vi "Process.vi"(8 "error in (no error)":errorcluster, 11 "SMO.UI":refnum<class "SMO.UI.lvclass">) -> (0 "error out":errorcluster, 3 "SMO.UI out":refnum<class "SMO.UI.lvclass">)   [LabVIEW 2021, in "smo.lvlib" / "SMO.UI.lvclass"]
uses:
  SMO.UI.lvclass
  C:/Repositories/SMO/src/SMO/SMO.lvclass
  SMO/Typedefs/Parent Call--Enum.ctl
  SMO/SMO.lvclass
  SMO/SMO.lvclass/SMO.ctl
  SMO.UI.lvclass/SMO.UI.ctl
  Typedefs/SMO.UI State--enum.ctl
  SMO/Private/GetVariant(Attr).vi
  Support/Attribute.Identity/Read UniqueName.vi
  Support/Attribute.Identity/Read Given Name.vi
  Support/Attribute.Identity/Read ProspectiveOwner.vi
  SMO/Private/ReftoDVR--SMO.vi
  SMO.UI.ReftoDVR.vi
  Support/Attribute.Identity/Attribute.Identity.lvclass
panel:
  in  "self terminate":bool
  out "Copyright":string="JKI State Machine Objects™\nhttp://jki.net/state-machine-objects/\nCopyright (C) 2005-2015, JKI <info@jki.net>\nALL RIGHTS RESERVED\n\nFor instructions on how to use the JKI State Machine Objects, examples and video tutorials, visit:\nhttp://jki.net/state-machine-objects/\n"
  # "JKI SMO UI"
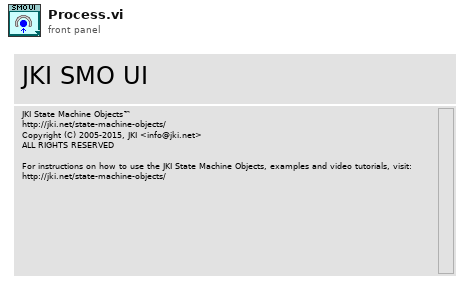
[diagram p1: front panel]
types:
  T1 = typedef "smo.lvlib/SMO.lvclass/Parent Call--Enum.ctl" = enum16{"Allows parent to run", "Does not request parent to run"}
  T2 = enum32{"invalid app kind", "Development System", "Run Time System", "Student Edition", "Embedded LabVIEW", "Evaluation", "Custom"}
  T3 = enum32{"Invalid", "Standard", "Closed", "Hidden", "Minimized", "Maximized"}
  T4 = typedef "smo.lvlib/SMO.UI.lvclass/SMO.UI State--enum.ctl" = enum16{"unknown", "Opened", "Closed"}
  T5 = cluster{"Core":cluster{"Current VI Reference":refnum<vi>, "Close Panel on Exit?":bool, "Last Error":cluster{"error":errorcluster, "previous state":string, "remaining states":string}}, "SMO out":refnum<class "SMO.UI.lvclass">}
  T6 = cluster{"Current VI Reference":refnum<vi>, "Close Panel on Exit?":bool, "Last Error":cluster{"error":errorcluster, "previous state":string, "remaining states":string}}
  T7 = typedef "smo.lvlib/SMO.lvclass/Protected Events.ctl" = cluster{"StopProcesses":refnum<user-event>, "AbortProcesses":refnum<user-event>, "Config Changed":refnum<user-event>, "Dependency":refnum<user-event>}
  T8 = typedef "smo.lvlib/SMO.UI.lvclass/PrivateEvents--Cluster.ctl" = cluster{"Show-Hide UI":refnum<user-event>}
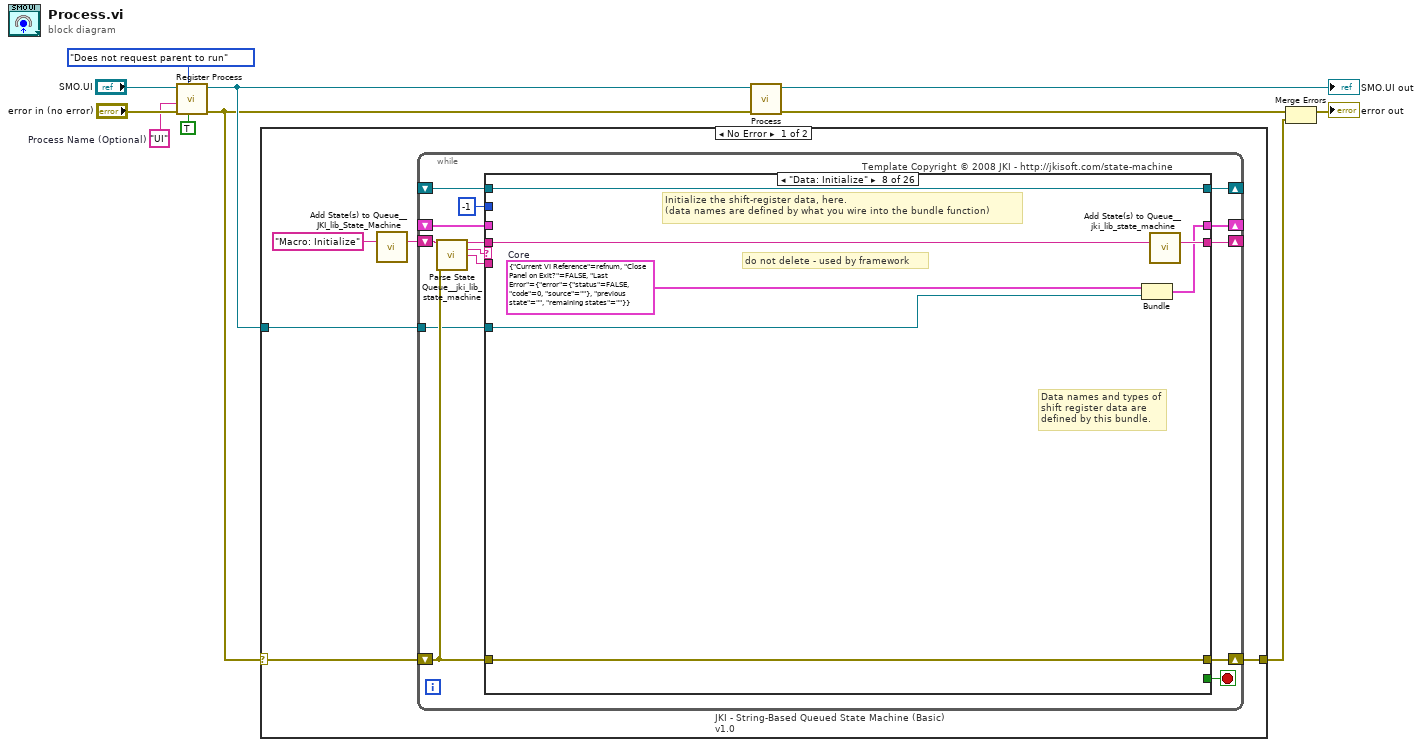
[diagram p0: block diagram]
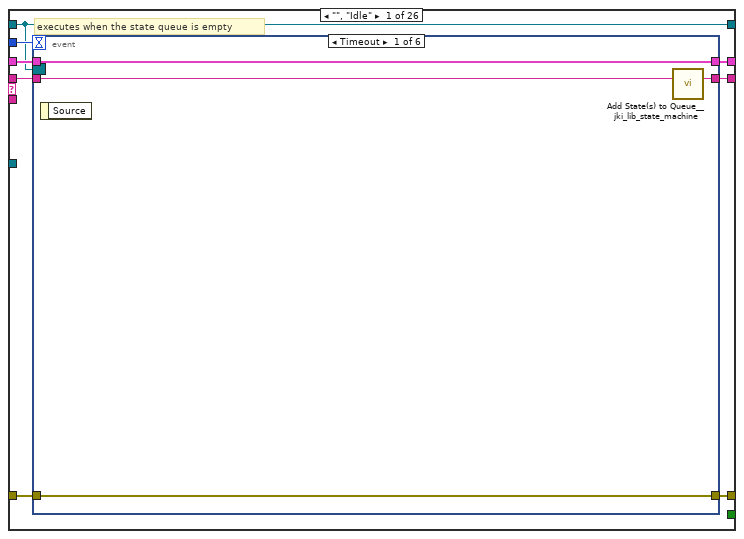
[diagram p2: hidden frame]
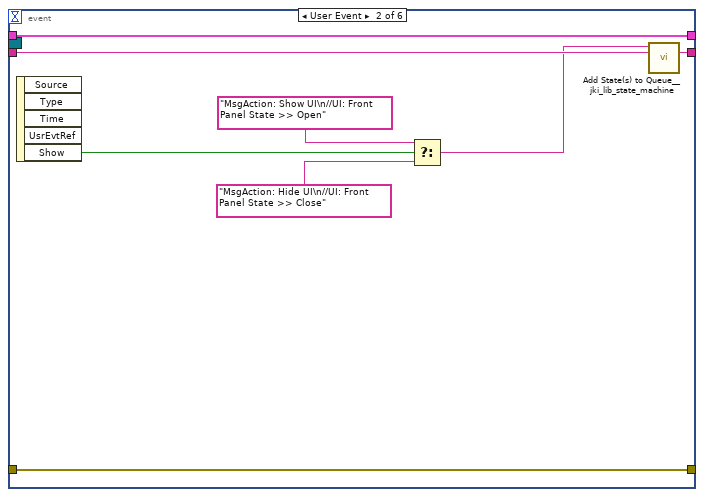
[diagram p3: hidden frame]
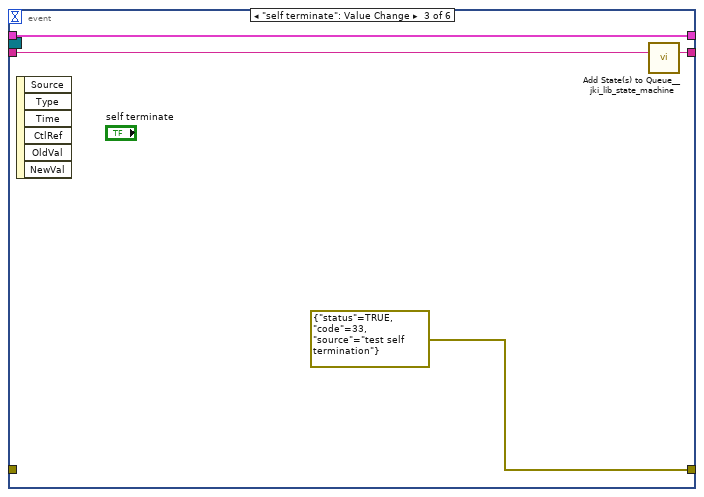
[diagram p4: hidden frame]
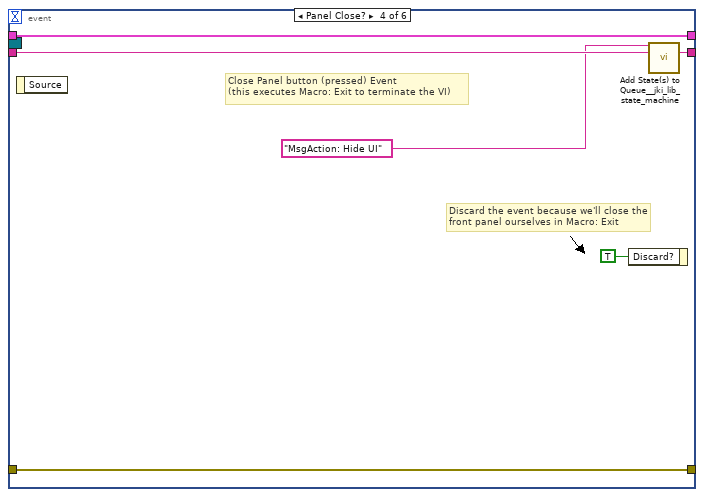
[diagram p5: hidden frame]
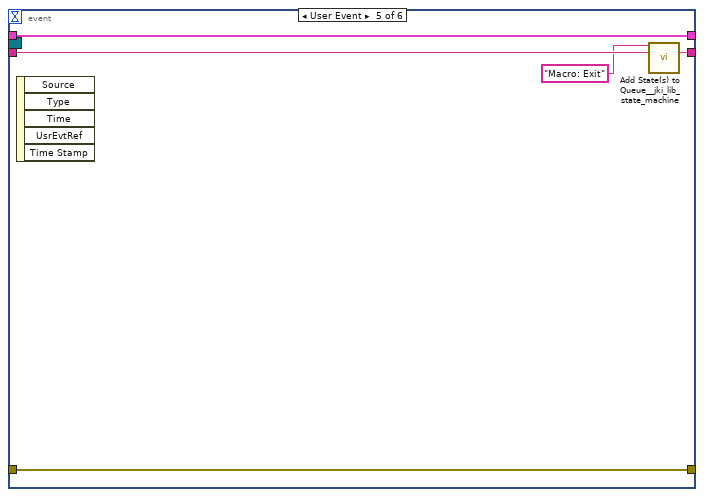
[diagram p6: hidden frame]
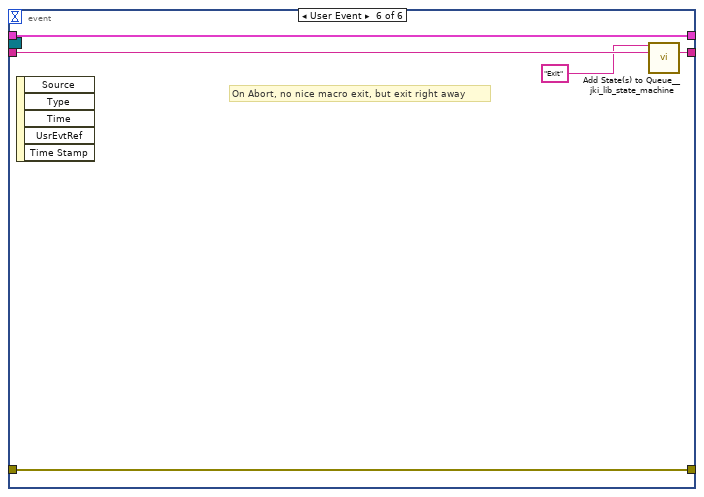
[diagram p7: hidden frame]
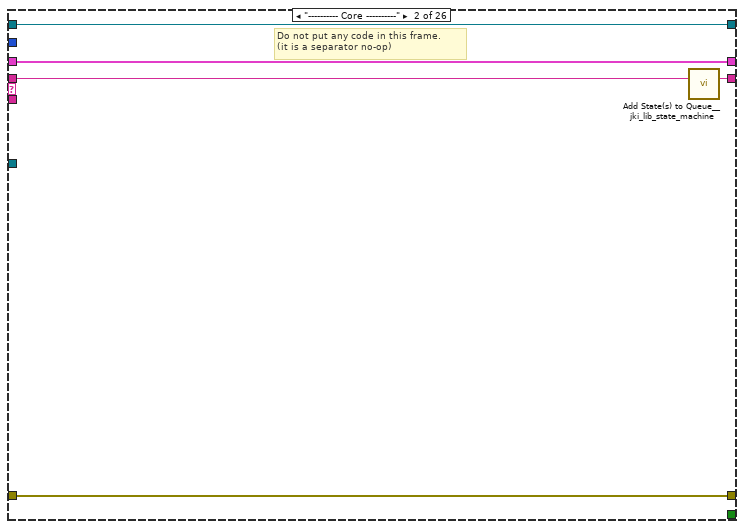
[diagram p8: hidden frame]
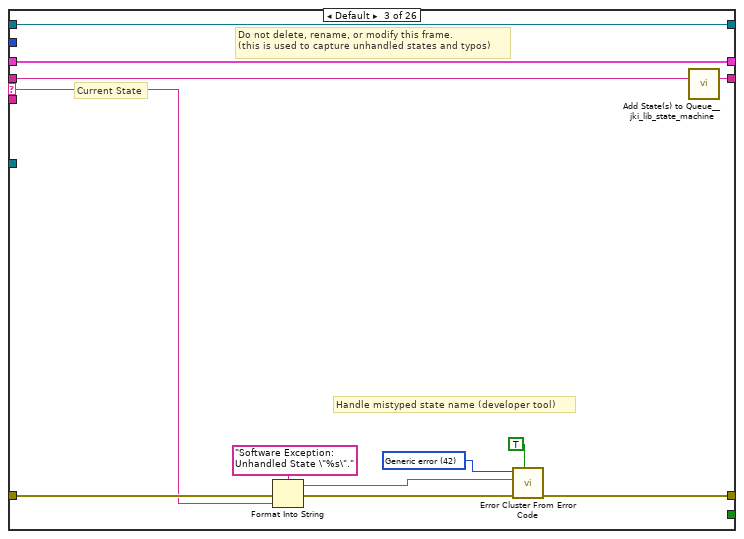
[diagram p9: hidden frame]
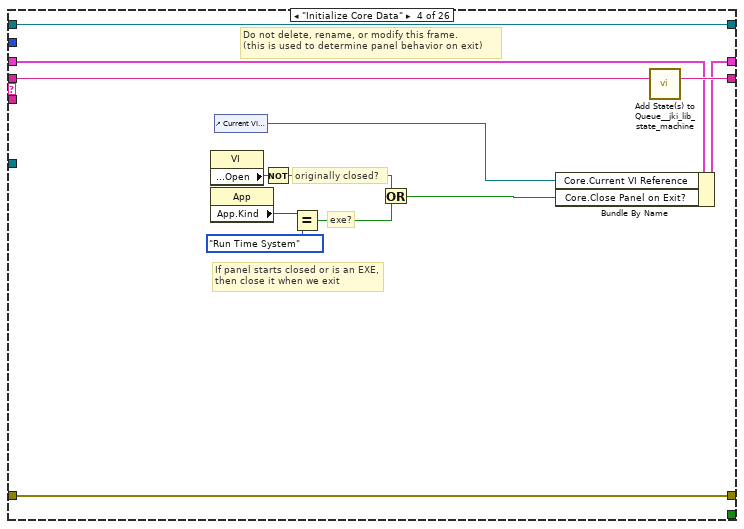
[diagram p10: hidden frame]
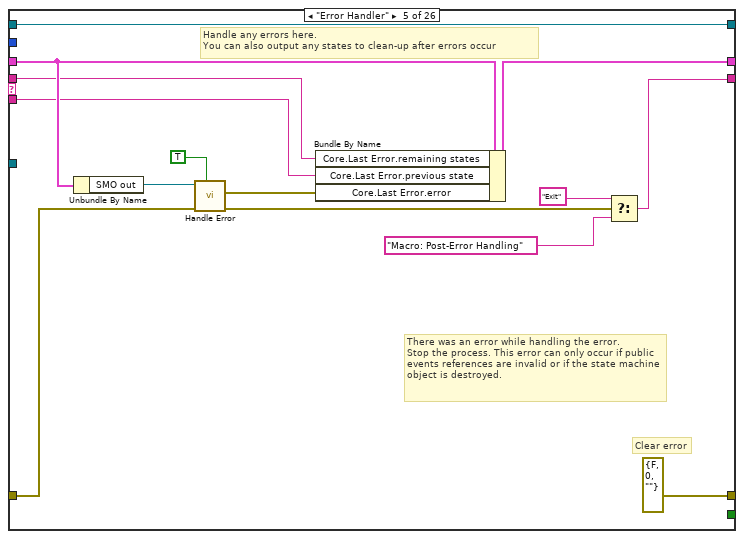
[diagram p11: hidden frame]
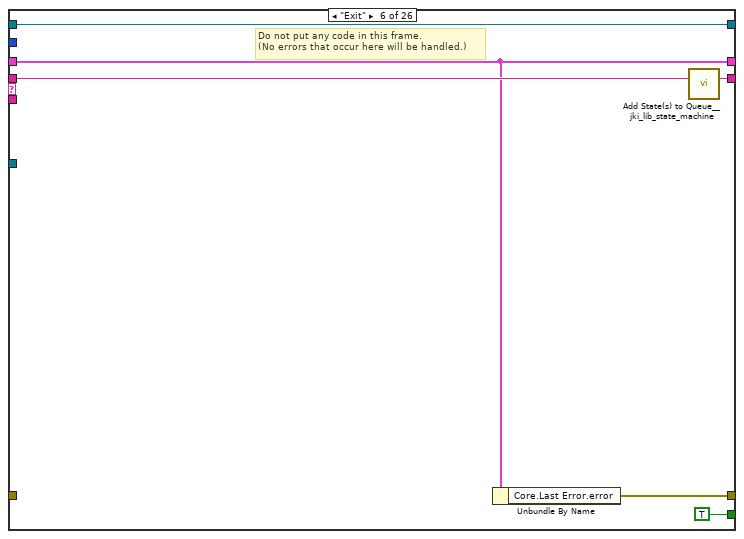
[diagram p12: hidden frame]
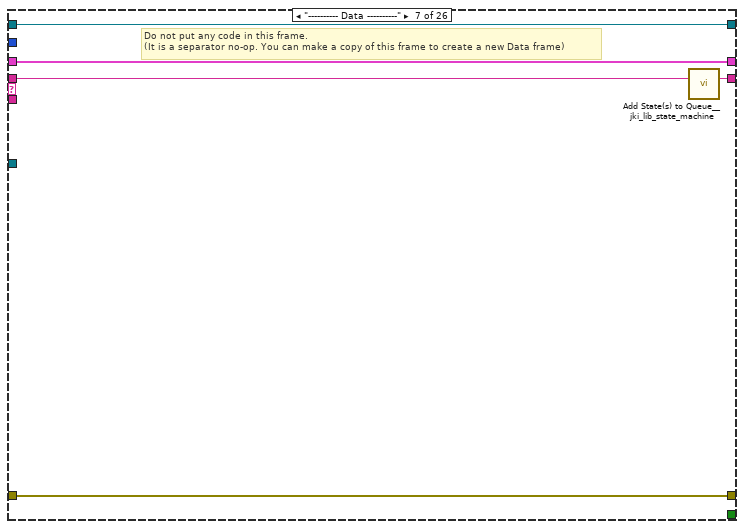
[diagram p13: hidden frame]
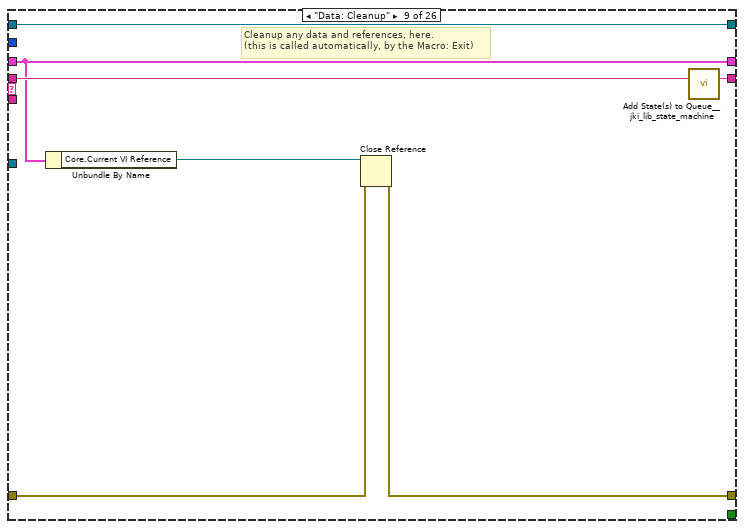
[diagram p14: hidden frame]
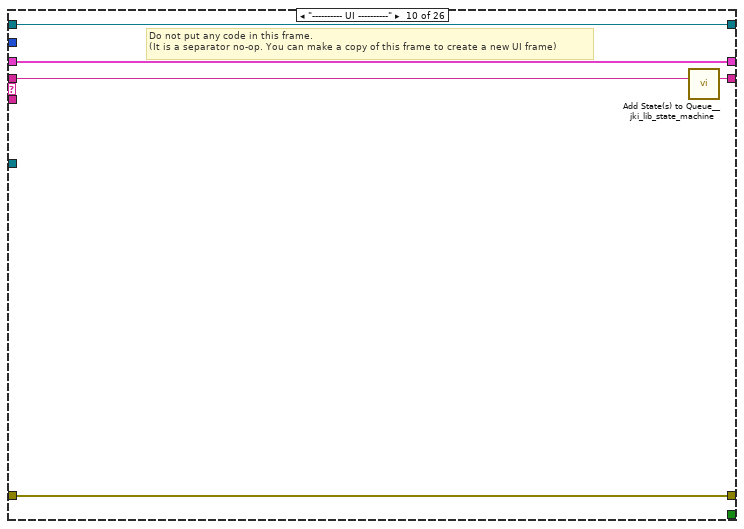
[diagram p15: hidden frame]
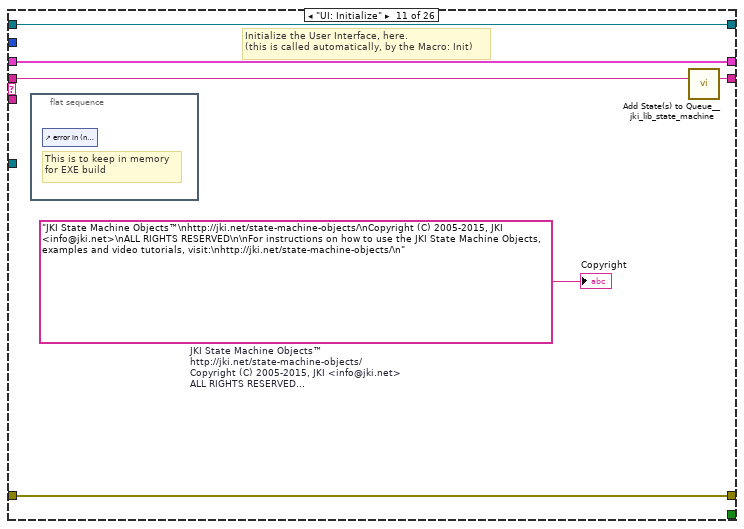
[diagram p16: hidden frame]
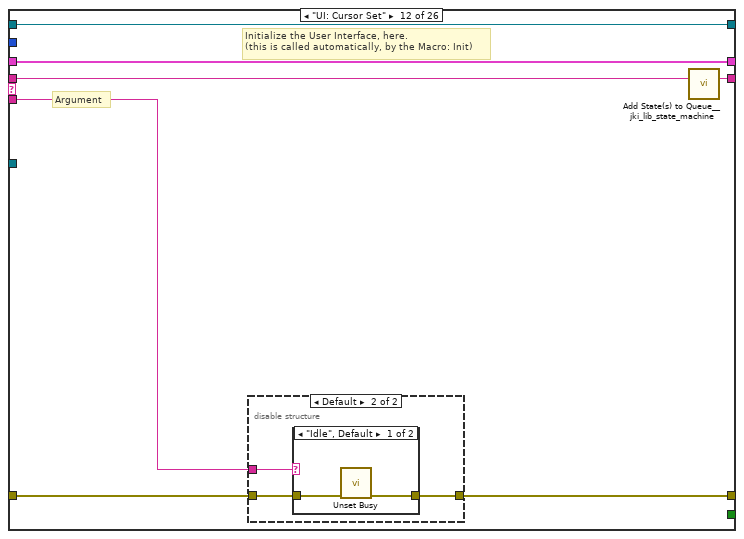
[diagram p17: hidden frame]
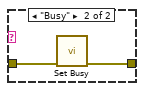
[diagram p19: hidden frame]
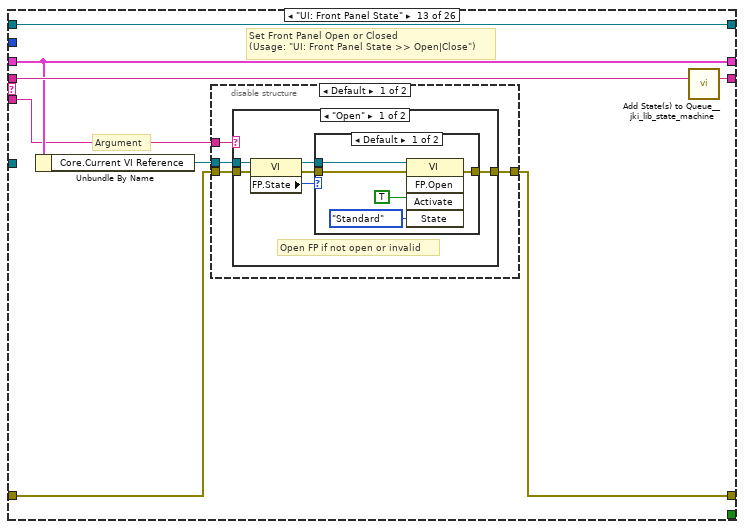
[diagram p20: hidden frame]
diagram:
  w4 = "UI"  # Process Name (Optional)
  n1 = call "Register Process.vi"("Forces Self to Run (F)"=TRUE, "Parent Call"=Parent_Call--Enum."Does not request parent to run", "error in (no error)"="error in (no error)", "Process Name (optional)"=w4, "SMO"="SMO.UI") -> ("error out"=w10:errorcluster, "SMO out"=w11:refnum<class "SMO.UI.lvclass">)  [unwired: 5 in]
  n2 = case shown="No Error" w10 {
    selector: w10 -> [w15 w324]
    tunnel: w11 -> [w16 _]
    tunnel: [w14 w324] -> w8
    frame No Error {
      n3 = call <vilib>:"Add State(s) to Queue__JKI_lib_State_Machine.vi"("State(s) in (\"\")"="Macro: Initialize") -> ("States Out"=w12:string)  [unwired: 14 in]
      n4 = while "JKI - String-Based Queued State Machine (Basic) v1.0" {
        shift-right: [w23] -> _
        shift-left: _ -> [w22]
        shift-right: [w26] -> w14
        shift-left: w15 -> [w20]
        shift-right: [w25] -> _
        shift-left: w12 -> [w27]
        tunnel: w16 -> [w19]
        shift-right: [w18] -> _
        shift-left: _ -> [w17]
        stop <- w24 stop-if-true
        # "Template Copyright © 2008 JKI - http://jkisoft.com/state-machine"
        n5 = call <vilib>:"Parse State Queue__jki_lib_state_machine.vi"("State Queue"=w27, "Error In (no error)"=w20) -> ("Remaining States"=w29:string, "Current State"=w30:string, "Arguments"=w28:string)  [unwired: 11 in]
        n6 = case shown="\"Data: Initialize\"" w30 {
          selector: w30 -> [_ _ w77 _ _ _ _ _ _ _ _ _ _ _ _ _ _ _ _ _ _ _ _ _ _ _]
          tunnel: w29 -> [w38 w75 w81 w100 w102 w120 w125 w132 w139 w144 w150 w157 w173 w205 w214 w223 w235 w240 w251 w263 w268 w280 w286 w291 w301 w316]
          tunnel: w28 -> [_ _ _ _ w103 _ _ _ _ _ _ w151 w169 _ _ _ _ _ _ _ _ _ _ _ _ _]
          tunnel: w22 -> [w36 w72 w79 w91 w112 w116 w122 _ w134 w141 w148 w155 w171 w202 w210 w219 w226 w237 w248 w260 w265 w278 w284 w288 w298 w313]
          tunnel: [w35 w73 w83 w97 errorcluster {"status"=FALSE, "code"=0, "source"=""} ("error out") w115 w123 w126 w135 w142 w147 w152 w166 w203 w212 w221 w233 w238 w242 w258 w266 w276 w282 w289 w292 w307] -> w26
          tunnel: w20 -> [w34 w73 w82 w97 w109 _ w123 w126 w136 w142 w147 w153 w167 w203 w212 w221 w233 w238 w243 w255 w266 w269 w282 w289 w296 w311]
          tunnel: [w37 w74 w80 w99 w101 w119 w124 w131 w138 w143 w149 w156 w172 w204 w213 w222 w234 w239 w250 w262 w267 w279 w285 w290 w300 w315] -> w25
          tunnel: [_ _ _ _ _ TRUE _ _ _ _ _ _ _ _ _ _ _ _ _ _ _ _ _ _ _ _] -> w24
          tunnel: [w33 w72 w79 w98 w111 w116 w122 w130 w134 w141 w148 w155 w171 w202 w210 w218 w226 w237 w248 w260 w265 w278 w284 w288 w298 w313] -> w23
          tunnel: -1 ("Timeout") -> [w32 _ _ _ _ _ _ _ _ _ _ _ _ _ _ _ _ _ _ _ _ _ _ _ _ _]
          tunnel: w19 -> [_ _ _ _ _ _ _ w127 _ _ _ _ _ _ _ _ _ _ _ _ _ _ _ _ _ _]
          tunnel: [w31 w71 w76 w88 w114 w117 w121 w129 w133 w140 w146 w154 w170 w201 w211 w220 w227 w236 w249 w261 w264 w275 w283 w287 w299 w314] -> w18
          tunnel: w17 -> [w31 w71 w76 w88 w114 w117 w121 w129 w133 w140 w146 w154 w170 w201 w211 w220 w227 w236 w249 w261 w264 _ w283 w287 w299 w314]
          frame "", "Idle" {
            # "executes when the state queue is empty"
            n7 = event shown="[0] Timeout" {
              selector: w31 -> [_ _ _ _ _ _]
              dyn-events: _ -> [_ _ _ _ _ _]
              timeout: w32 -> [_ _ _ _ _ _]
              tunnel: w38 -> [w42 w50 w54 w60 w65 w70]
              tunnel: [w41 w49 w53 w59 w64 w69] -> w37
              tunnel: w36 -> [w39 w47 w52 w56 w62 w67]
              tunnel: [w40 w48 errorcluster {"status"=TRUE, "code"=33, "source"="test self termination"} ("error IO") w58 w63 w68] -> w35
              tunnel: w34 -> [w40 w48 _ w58 w63 w68]
              tunnel: [w39 w47 w52 w56 w62 w67] -> w33
              event Timeout {
                n8 = event-data() -> ()  [unwired: 1 in, 1 out]
                n9 = call <vilib>:"Add State(s) to Queue__jki_lib_state_machine.vi"("State(s) in (\"\")"=w42) -> ("States Out"=w41:string)  [unwired: 14 in]
              }
              event User Event {
                n10 = event-data() -> ("Show"=w46:bool)  [unwired: 1 in, 4 out]
                n11 = Select(t="MsgAction: Show UI\n//UI: Front Panel State >> Open" ("State(s) in Front (\"\")"), s=w46, f="MsgAction: Hide UI\n//UI: Front Panel State >> Close" ("State(s) in Front (\"\")")) -> (s? t:f=w43:string)
                n12 = call <vilib>:"Add State(s) to Queue__jki_lib_state_machine.vi"("State(s) in Front (\"\")"=w43, "State(s) in (\"\")"=w50) -> ("States Out"=w49:string)  [unwired: 13 in]
              }
              event "self terminate": Value Change {
                n13 = event-data() -> ()  [unwired: 1 in, 6 out]
                n14 = call <vilib>:"Add State(s) to Queue__jki_lib_state_machine.vi"("State(s) in (\"\")"=w54) -> ("States Out"=w53:string)  [unwired: 14 in]
              }
              event Panel Close? {
                # "Discard the event because we'll close the front panel ourselves in Macro: Exit"
                # "Close Panel button (pressed) Event\n(this executes Macro: Exit to terminate the VI)"
                n15 = event-data() -> ()  [unwired: 1 in, 1 out]
                n16 = event-data("Discard?"=TRUE) -> ()  [unwired: 1 in, 1 out]
                n17 = call <vilib>:"Add State(s) to Queue__jki_lib_state_machine.vi"("State(s) in Front (\"\")"="MsgAction: Hide UI", "State(s) in (\"\")"=w60) -> ("States Out"=w59:string)  [unwired: 13 in]
              }
              event User Event {
                n18 = event-data() -> ()  [unwired: 1 in, 5 out]
                n19 = call <vilib>:"Add State(s) to Queue__jki_lib_state_machine.vi"("State(s) in Front (\"\")"="Macro: Exit", "State(s) in (\"\")"=w65) -> ("States Out"=w64:string)  [unwired: 13 in]
              }
              event User Event {
                # "On Abort, no nice macro exit, but exit right away"
                n20 = event-data() -> ()  [unwired: 1 in, 5 out]
                n21 = call <vilib>:"Add State(s) to Queue__jki_lib_state_machine.vi"("State(s) in Front (\"\")"="Exit", "State(s) in (\"\")"=w70) -> ("States Out"=w69:string)  [unwired: 13 in]
              }
            }
          }
          frame "---------- Core ----------" {
            # "Do not put any code in this frame.\n(it is a separator no-op)"
            n22 = call <vilib>:"Add State(s) to Queue__jki_lib_state_machine.vi"("State(s) in (\"\")"=w75) -> ("States Out"=w74:string)  [unwired: 14 in]
          }
          frame Default {
            w86 = 42 items=["No error", "Argument error", "Memory is full", "Out of zone", "End of file", "File already open", "Generic file I/O error", "File not found", "File permission error", "Disk is full", "Duplicate path", "Too many files open", "System feature not enabled", "Resource file not found", "Cannot add resource", "Resource not found", "Image not found", "Image memory error", "Pen does not exist", "Config type invalid", "Config token not found", "Config parse error", "Config memory error", "Bad external code format", "Bad external code offset", "External code not present", "Null window", "Destroy window error", "Null menu", "Print aborted", "Bad print record", "Print driver error", "Windows error during printing", "Memory error during printing", "Print dialog error", "Generic print error", "Invalid device refnum", "Device not found", "Device parameter error", "Device unit error", "Cannot open device", "Device call aborted", "Generic error", "Cancelled by user", "Object ID too low", "Object ID too high", "Object not in heap", "Unknown heap", "Unknown object (invalid DefProc)", "Unknown object (DefProc not in table)", "Message out of range", "Invalid (null) method", "Unknown message", "Manager call not supported", "Bad address", "Network operation in progress", "Network operation timed out", "Connection is busy", "Network attribute not supported", "Network error", "Address in use", "System out of memory", "Connection aborted", "Connection refused", "Not connected", "Already connected", "Connection closed", "Initialization error (interapplication manager)", "Bad occurrence", "Wait on unbound occurrence handler", "Occurrence queue overflow", "Datalog type conflict", "Unused", "Unrecognized type (interapplication manager)", "Memory corrupt", "Failed to make temporary DLL", "Old CIN version", "Drag socket not found", "Failed to load drop-object", "Failed to register OLE object", "Failed to release OLE object", "Format specifier type mismatch", "Unknown format specifier", "Too few format specifiers", "Too many format specifiers", "Scan failed", "Newer CIN version", "Error converting to variant", "Runtime menu error", "Password tampered", "Variant attribute not found", "Incompatible variant data type", "Event data is not available", "Event Store is not present", "Occurrence is not found", "Event Queue is not created", "Event info is not available", "Refnum passed is NULL", "Error retrieving Class GUID", "Error retrieving CoClass GUID", "Error retrieving TypeLib GUID.", "Bad built application magic bytes.", "Specific driver is different from the specific driver associated with the Logical Name.", "There is no session opened to the class driver.", "Max Error", "MAX - Error with config objects", "MAX - Error loading configuration", "MAX - Group not supported"]
            # "Current State"
            # "Do not delete, rename, or modify this frame.\n(this is used to capture unhandled states and typos)"
            # "Handle mistyped state name (developer tool)"
            n23 = Format Into String(format string="Software Exception: Unhandled State \"%s\"." ("message"), error in=w82, w77) -> (resulting string=w85:string, error out=w84:errorcluster)  [unwired: 1 in]
            n24 = call <vilib>:"Error Cluster From Error Code.vi"("show call chain? (False)"=TRUE, "error in (no error)"=w84, "error message (\"\")"=w85, "error code (0)"=w86) -> ("error out"=w83:errorcluster)  [unwired: 5 in]
            n25 = call <vilib>:"Add State(s) to Queue__jki_lib_state_machine.vi"("State(s) in (\"\")"=w81) -> ("States Out"=w80:string)  [unwired: 14 in]
          }
          frame "Initialize Core Data" {
            # "Do not delete, rename, or modify this frame.\n(this is used to determine panel behavior on exit)"
            # "originally closed?"
            # "exe?"
            # "If panel starts closed or is an EXE, then close it when we exit"
            n26 = property class="VI"() -> ("Front Panel.Open"=w96:bool)  [unwired: 2 in, 2 out]
            n27 = property class="App"() -> ("App.Kind"=w95:T2)  [unwired: 2 in, 2 out]
            n28 = control-ref of="Current VI Reference"() -> (w89:refnum<vi>)
            n29 = Not(x=w96) -> (.not. x?=w93:bool)
            n30 = Equal?(x=w95, y=T2."Run Time System" ("Application:Kind")) -> (x = y?=w92:bool)
            n31 = Or(x=w93, y=w92) -> (x .or. y?=w90:bool)
            n32 = Bundle By Name(cluster=w91, "Core.Current VI Reference"=w89, "Core.Close Panel on Exit?"=w90) -> (w98:T5)
            n33 = call <vilib>:"Add State(s) to Queue__jki_lib_state_machine.vi"("State(s) in (\"\")"=w100) -> ("States Out"=w99:string)  [unwired: 14 in]
          }
          frame "Error Handler" {
            # "There was an error while handling the error.\nStop the process. This error can only occur if public events references are invalid or if the state machine object is destroyed."
            # "Handle any errors here.\nYou can also output any states to clean-up after errors occur"
            # "Clear error"
            n34 = Unbundle By Name(w112) -> ("SMO out"=w113:refnum<class "SMO.UI.lvclass">)
            n35 = call-dynamic "Handle Error.vi"("Stop on Unhandled Error (T)"=TRUE, "error in"=w109, "SMO"=w113) -> ("handling error"=w107:errorcluster, "Unhandled error"=w110:errorcluster)  [unwired: 6 in, 1 out]
            n36 = Bundle By Name(cluster=w112, "Core.Last Error.remaining states"=w102, "Core.Last Error.previous state"=w103, "Core.Last Error.error"=w110) -> (w111:T5)
            n37 = Select(t="Exit", s=w107, f="Macro: Post-Error Handling") -> (s? t:f=w101:string)
          }
          frame "Exit" {
            # "Do not put any code in this frame.\n(No errors that occur here will be handled.)"
            n38 = Unbundle By Name(w116) -> ("Core.Last Error.error"=w115:errorcluster)
            n39 = call <vilib>:"Add State(s) to Queue__jki_lib_state_machine.vi"("State(s) in (\"\")"=w120) -> ("States Out"=w119:string)  [unwired: 14 in]
          }
          frame "---------- Data ----------" {
            # "Do not put any code in this frame.\n(It is a separator no-op. You can make a copy of this frame to create a new Data frame)"
            n40 = call <vilib>:"Add State(s) to Queue__jki_lib_state_machine.vi"("State(s) in (\"\")"=w125) -> ("States Out"=w124:string)  [unwired: 14 in]
          }
          frame "Data: Initialize" {
            w128 = T6 {"Current VI Reference"=refnum, "Close Panel on Exit?"=FALSE, "Last Error"={"error"={"status"=FALSE, "code"=0, "source"=""}, "previous state"="", "remaining states"=""}}  # Core
            # "do not delete - used by framework"
            # "Data names and types of shift register data are defined by this bundle."
            # "Initialize the shift-register data, here.\n(data names are defined by what you wire into the bundle function)"
            n41 = Bundle("Core"=w128, "SMO out"=w127) -> (w130:T5)  [unwired: 1 in]
            n42 = call <vilib>:"Add State(s) to Queue__jki_lib_state_machine.vi"("State(s) in (\"\")"=w132) -> ("States Out"=w131:string)  [unwired: 14 in]
          }
          frame "Data: Cleanup" {
            # "Cleanup any data and references, here.\n(this is called automatically, by the Macro: Exit)"
            n43 = Unbundle By Name(w134) -> ("Core.Current VI Reference"=w137:refnum<vi>)
            n44 = Close Reference(reference=w137, error in (no error)=w136) -> (error out=w135:errorcluster)
            n45 = call <vilib>:"Add State(s) to Queue__jki_lib_state_machine.vi"("State(s) in (\"\")"=w139) -> ("States Out"=w138:string)  [unwired: 14 in]
          }
          frame "---------- UI ----------" {
            # "Do not put any code in this frame.\n(It is a separator no-op. You can make a copy of this frame to create a new UI frame)"
            n46 = call <vilib>:"Add State(s) to Queue__jki_lib_state_machine.vi"("State(s) in (\"\")"=w144) -> ("States Out"=w143:string)  [unwired: 14 in]
          }
          frame "UI: Initialize" {
            w145 = "JKI State Machine Objects™\nhttp://jki.net/state-machine-objects/\nCopyright (C) 2005-2015, JKI <info@jki.net>\nALL RIGHTS RESERVED\n\nFor instructions on how to use the JKI State Machine Objects, examples and video tutorials, visit:\nhttp://jki.net/state-machine-objects/\n"  # JKI State Machine Objects™ http://jki.net/state-machine-objects/ Copyright (C) 2005-2015, JKI <info@jki.net> ALL RIGHTS RESERVED  For instructions on how to use the JKI State Machine Objects, examples and video tutorials, visit: http://jki.net/state-machine-objects/
            # "Initialize the User Interface, here.\n(this is called automatically, by the Macro: Init)"
            n47 = flat-sequence {
              frame #0 {
                # "This is to keep in memory\nfor EXE build"
                n48 = control-ref of="error in (no error)"() -> ()  [unwired: 1 out]
              }
            }
            n49 = call <vilib>:"Add State(s) to Queue__jki_lib_state_machine.vi"("State(s) in (\"\")"=w150) -> ("States Out"=w149:string)  [unwired: 14 in]
            "Copyright" <- w145
          }
          frame "UI: Cursor Set" {
            # "Argument"
            # "Initialize the User Interface, here.\n(this is called automatically, by the Macro: Init)"
            n50 = disable-structure shown="Default" {
              disable-tunnel: w153 -> [w158 w161]
              disable-tunnel: [w158 w160] -> w152
              disable-tunnel: w151 -> [_ w159]
              frame condition #0 {
              }
              frame condition #1 (active) {
                n51 = case shown="\"Idle\", Default" w159 {
                  tunnel: w161 -> [w163 w165]
                  tunnel: [w162 w164] -> w160
                  frame "Idle", Default {
                    n52 = call <vilib>:"Unset Busy.vi"("error in (no error)"=w163) -> ("error out"=w162:errorcluster)  [unwired: 10 in]
                  }
                  frame "Busy" {
                    n53 = call <vilib>:"Set Busy.vi"("error in (no error)"=w165) -> ("error out"=w164:errorcluster)  [unwired: 9 in, 1 out]
                  }
                }
              }
            }
            n54 = call <vilib>:"Add State(s) to Queue__jki_lib_state_machine.vi"("State(s) in (\"\")"=w157) -> ("States Out"=w156:string)  [unwired: 14 in]
          }
          frame "UI: Front Panel State" {
            # "Argument"
            # "Set Front Panel Open or Closed\n(Usage: \"UI: Front Panel State >> Open|Close\")"
            n55 = Unbundle By Name(w171) -> ("Core.Current VI Reference"=w168:refnum<vi>)
            n56 = disable-structure shown="Default" {
              disable-tunnel: w167 -> [w177 w200]
              disable-tunnel: [w176 w200] -> w166
              disable-tunnel: w168 -> [w175 _]
              disable-tunnel: w169 -> [w174 _]
              frame condition #0 (active) {
                n57 = case shown="\"Open\"" w174 {
                  tunnel: w177 -> [w181 w194]
                  tunnel: [w183 w195] -> w176
                  tunnel: w175 -> [w182 w192]
                  frame "Open" {
                    # "Open FP if not open or invalid"
                    n58 = property class="VI"(reference=w182, error in=w181) -> (reference out=w179:refnum<vi>, error out=w180:errorcluster, "FP.State"=w178:T3)
                    n59 = case shown="Default" w178 {
                      tunnel: [w186 w189] -> w183
                      tunnel: w180 -> [w185 w189]
                      tunnel: w179 -> [w184 _]
                      frame Default {
                        n60 = invoke class="VI" method="FP.Open"(reference=w184, error in=w185, "Activate"=TRUE, "State"=T3."Standard") -> (error out=w186:errorcluster)  [unwired: 1 in, 4 out]
                      }
                      frame "Invalid", "Standard" {
                      }
                    }
                  }
                  frame "Close", Default {
                    # "Close FP is not Closed or Invalid"
                    n61 = property class="VI"(reference=w192, error in=w194) -> (reference out=w191:refnum<vi>, error out=w193:errorcluster, "FP.State"=w190:T3)
                    n62 = case shown="Default" w190 {
                      tunnel: [w196 w199] -> w195
                      tunnel: w193 -> [w196 w198]
                      tunnel: w191 -> [_ w197]
                      frame "Invalid", "Closed" {
                      }
                      frame Default {
                        n63 = invoke class="VI" method="FP.Close"(reference=w197, error in=w198) -> (error out=w199:errorcluster)  [unwired: 1 in, 2 out]
                      }
                    }
                  }
                }
              }
              frame condition #1 {
              }
            }
            n64 = call <vilib>:"Add State(s) to Queue__jki_lib_state_machine.vi"("State(s) in (\"\")"=w173) -> ("States Out"=w172:string)  [unwired: 14 in]
          }
          frame "---------- Macro ----------" {
            # "Do not put any code in this frame.\n(It is a separator no-op. You can make a copy of this frame to create a new Macro frame)"
            n65 = call <vilib>:"Add State(s) to Queue__jki_lib_state_machine.vi"("State(s) in (\"\")"=w205) -> ("States Out"=w204:string)  [unwired: 14 in]
          }
          frame "Macro: Initialize" {
            w208 = "UI: Initialize\n//UI: Front Panel State >> Open\n\n//Test: Start SMO Dependency //Only for development purpose."  # UI: Initialize //UI: Front Panel State >> Open  //Test: Start SMO Dependency //Only for development purpose.
            # "Initialization Macro\n(This is called once, when the VI starts)"
            n66 = call <vilib>:"Add State(s) to Queue__jki_lib_state_machine.vi"("State(s) in Front (\"\")"="Data: Initialize\nInitialize Core Data\nEvents: Register", "State(s) in (\"\")"="Process: Sync", "State(s) at Back (\"\")"=w208) -> ("States Out"=w207:string)  [unwired: 12 in]
            n67 = call <vilib>:"Add State(s) to Queue__jki_lib_state_machine.vi"("State(s) in Front (\"\")"=w207, "State(s) in (\"\")"=w214) -> ("States Out"=w213:string)  [unwired: 13 in]
          }
          frame "Macro: Post-Error Handling" {
            # "Clear Last Error?"
            n68 = Unbundle By Name(w219) -> ("Core.Last Error.error"=w217:errorcluster)  [unwired: 2 out]
            n69 = case shown="False" FALSE {
              tunnel: w217 -> [w224 _]
              tunnel: [w224 _] -> w216
              frame False {
              }
              frame True {
              }
            }
            n70 = Bundle By Name(cluster=w219, "Core.Last Error.error"=w216) -> (w218:T5)
            n71 = call <vilib>:"Add State(s) to Queue__jki_lib_state_machine.vi"("State(s) in (\"\")"=w223) -> ("States Out"=w222:string)  [unwired: 14 in]
          }
          frame "Macro: Exit" {
            # "Exit Macro\n(This is called once, when the VI exits)"
            n72 = Unbundle By Name(w226) -> ("Core.Close Panel on Exit?"=w232:bool)
            n73 = Select(t="UI: Front Panel State >> Close", s=w232, f="") -> (s? t:f=w229:string)
            n74 = call <vilib>:"Add State(s) to Queue__jki_lib_state_machine.vi"("State(s) in (\"\")"=w229, "State(s) at Back (\"\")"="Data: Cleanup\nEvents: Unregister\nProcess: Sync\nExit") -> ("States Out"=w228:string)  [unwired: 13 in]
            n75 = call <vilib>:"Add State(s) to Queue__jki_lib_state_machine.vi"("State(s) in Front (\"\")"=w228, "State(s) in (\"\")"=w235) -> ("States Out"=w234:string)  [unwired: 13 in]
          }
          frame "---------- Process ----------" {
            # "Template Separator\n(You can make a copy of, or modify, this frame)"
            n76 = call <vilib>:"Add State(s) to Queue__jki_lib_state_machine.vi"("State(s) in (\"\")"=w240) -> ("States Out"=w239:string)  [unwired: 14 in]
          }
          frame "Process: Sync" {
            n77 = Unbundle By Name(w248) -> ("SMO out"=w244:refnum<class "SMO.UI.lvclass">)
            n78 = call "WaitOnProcessSync.vi"("error in (no error)"=w243, "SMO"=w244) -> ("error out"=w242:errorcluster, "Don't run?"=w247:bool)  [unwired: 7 in, 1 out]
            n79 = Select(t="Data: Cleanup\nEvents: Unregister\nExit", s=w247, f="") -> (s? t:f=w241:string)
            n80 = call <vilib>:"Add State(s) to Queue__jki_lib_state_machine.vi"("State(s) in Front (\"\")"=w241, "State(s) in (\"\")"=w251) -> ("States Out"=w250:string)  [unwired: 13 in]
          }
          frame "Test: Start SMO Dependency" {
            # ">> Returns the instance of \"Dummy\"\nand ignores the other levels dependencies"
            n81 = Unbundle By Name(w260) -> ("SMO out"=w259:refnum<class "SMO.UI.lvclass">)
            n82 = call "LaunchDependency.vi"("error in (no error)"=w255, "Dependency Name"="Dummy", "Dependency Type"=refnum<class "SMO.lvclass"> refnum ("SMO.lvclass"), "SMO in"=w259) -> ("error out"=w258:errorcluster, "SMO in"=w252:refnum<class "SMO.UI.lvclass">)  [unwired: 4 in, 2 out]
            n83 = call "ListThisLevelDependencies.vi"("SMO in"=w252) -> ("[My Dependencies]"=w254:refnum<class "SMO.lvclass">[])  [unwired: 8 in, 2 out]
            n84 = Index Array(array=w254) -> (element=w253:refnum<class "SMO.lvclass">)  [unwired: 1 in]
            n85 = call "Get Name.vi"("SMO"=w253) -> ()  [unwired: 6 in, 5 out]
            n86 = call <vilib>:"Add State(s) to Queue__jki_lib_state_machine.vi"("State(s) in (\"\")"=w263) -> ("States Out"=w262:string)  [unwired: 14 in]
          }
          frame "---------- Events ----------" {
            # "Template Separator\n(You can make a copy of, or modify, this frame)"
            n87 = call <vilib>:"Add State(s) to Queue__jki_lib_state_machine.vi"("State(s) in (\"\")"=w268) -> ("States Out"=w267:string)  [unwired: 14 in]
          }
          frame "Events: Register" {
            n88 = Unbundle By Name(w278) -> ("SMO out"=w274:refnum<class "SMO.UI.lvclass">)
            n89 = call "GetProtectedEvents.vi"("error in (no error)"=w269, "SMO"=w274) -> ("error out"=w270:errorcluster, "SMO Protected Events"=w277:T7, "SMO"=w271:refnum<class "SMO.UI.lvclass">)  [unwired: 7 in]
            n90 = call "SMO.UI.GetPrivateEvents.vi"("error in (no error)"=w270, "SMO.UI"=w271) -> ("error out"=w272:errorcluster, "SMO.UI Private Events"=w273:T8)  [unwired: 7 in, 1 out]
            n91 = register-events(error in=w272, w277, w273) -> (reference out=w275:refnum<event-registration>, error out=w276:errorcluster)  [unwired: 1 in]
            n92 = call <vilib>:"Add State(s) to Queue__jki_lib_state_machine.vi"("State(s) in (\"\")"=w280) -> ("States Out"=w279:string)  [unwired: 14 in]
          }
          frame "Events: Unregister" {
            # "Your code here.\n(You can make a copy of, or modify, this frame)"
            n93 = Unregister For Events(event registration refnum=w283, error in=w282) -> (error out=w281:errorcluster)
            n94 = call <vilib>:"Clear Errors.vi"("error in (no error)"=w281) -> ()  [unwired: 5 in, 2 out]
            n95 = call <vilib>:"Add State(s) to Queue__jki_lib_state_machine.vi"("State(s) in (\"\")"=w286) -> ("States Out"=w285:string)  [unwired: 14 in]
          }
          frame "---------MsgAction---------" {
            # "MsgAction Separator\n(You can make a copy of, or modify, this frame)"
            n96 = call <vilib>:"Add State(s) to Queue__jki_lib_state_machine.vi"("State(s) in (\"\")"=w291) -> ("States Out"=w290:string)  [unwired: 14 in]
          }
          frame "MsgAction: Show UI" {
            n97 = Unbundle By Name(w298) -> ("SMO out"=w297:refnum<class "SMO.UI.lvclass">)
            n98 = call-dynamic "Show User Interface.vi"("error in (no error)"=w296, "Show UI"=TRUE, "SMO.UI"=w297) -> ("error out"=w293:errorcluster, "SMO.UI out"=w294:refnum<class "SMO.UI.lvclass">)  [unwired: 7 in]
            n99 = case shown="No Error" w293 {
              selector: w293 -> [w304 w306]
              tunnel: w294 -> [w305 _]
              tunnel: [w303 w306] -> w292
              frame No Error {
                n100 = call "NotifyUIState.vi"("error in (no error)"=w304, "UI State"=SMO.UI_State--enum."Opened", "SMO.UI"=w305) -> ("error out"=w303:errorcluster)  [unwired: 7 in, 1 out]
              }
              frame Error {
              }
            }
            n101 = call <vilib>:"Add State(s) to Queue__jki_lib_state_machine.vi"("State(s) in (\"\")"=w301) -> ("States Out"=w300:string)  [unwired: 14 in]
          }
          frame "MsgAction: Hide UI" {
            n102 = Unbundle By Name(w313) -> ("SMO out"=w312:refnum<class "SMO.UI.lvclass">)
            n103 = call-dynamic "Show User Interface.vi"("error in (no error)"=w311, "Show UI"=FALSE, "SMO.UI"=w312) -> ("error out"=w308:errorcluster, "SMO.UI out"=w309:refnum<class "SMO.UI.lvclass">)  [unwired: 7 in]
            n104 = case shown="No Error" w308 {
              selector: w308 -> [w321 w323]
              tunnel: w309 -> [w322 _]
              tunnel: [w317 w323] -> w307
              frame No Error {
                n105 = call "NotifyUIHidden.vi"("error in (no error)"=w321, "SMO.UI"=w322) -> ("error out"=w318:errorcluster, "SMO.UI out"=w319:refnum<class "SMO.UI.lvclass">)  [unwired: 8 in]
                n106 = call "NotifyUIState.vi"("error in (no error)"=w318, "UI State"=SMO.UI_State--enum."Closed", "SMO.UI"=w319) -> ("error out"=w317:errorcluster)  [unwired: 7 in, 1 out]
              }
              frame Error {
              }
            }
            n107 = call <vilib>:"Add State(s) to Queue__jki_lib_state_machine.vi"("State(s) in (\"\")"=w316) -> ("States Out"=w315:string)  [unwired: 14 in]
          }
        }
      }
    }
    frame Error {
    }
  }
  n108 = call-parent "Process.vi"("error in"=w10, "SMO"=w11) -> ("error out"=w9:errorcluster, "SMO out"=→"SMO.UI out":refnum<class "SMO.UI.lvclass">)  [unwired: 8 in]
  n109 = Merge Errors(w9, w8) -> (→"error out":errorcluster)
